vi "Setup.vi"(11 "Test Framework.lvclass":refnum<class "Test Framework.lvclass">) -> (0 "Error Out":errorcluster, 3 "Test Framework.lvclass Out":refnum<class "Test Framework.lvclass">)   [LabVIEW 2020, in "Test Framework.lvclass"]
uses:
  Test Framework.lvclass
  Path Control/PathControl.lvclass
  Instruments/Temperature Control/Temperature Control.lvclass
  Instruments/Power Supply/Power Supply.lvclass
  XML Handler/XML Handler.lvclass
  Test Framework.lvclass/Test Framework.ctl
  <vilib>/Utility/xml.llb/Read From XML File(string).vi
  Devices/Device.lvclass
  Measurements/Measurement.lvclass
panel:
  out "Available devices":string[](array[string])
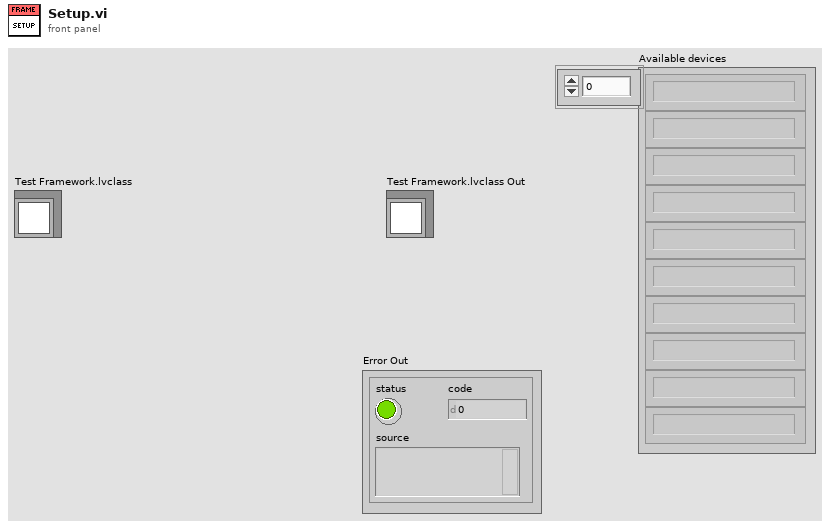
[diagram p1: front panel]
types:
  T1 = cluster{"Restart?":bool, "User system setting file":path}
  T2 = typedef "Device.lvclass/Device Information Cluster.ctl" = cluster{"Device Info":string[][], "Default Values":T3[], "Fetched info":string[][]}
  T3 = typedef "PIC-Device.lvclass/Register to Write.ctl" = cluster{"Register":u32, "Value":u32, "Dev Address":u32, "Physical Adress":u32}
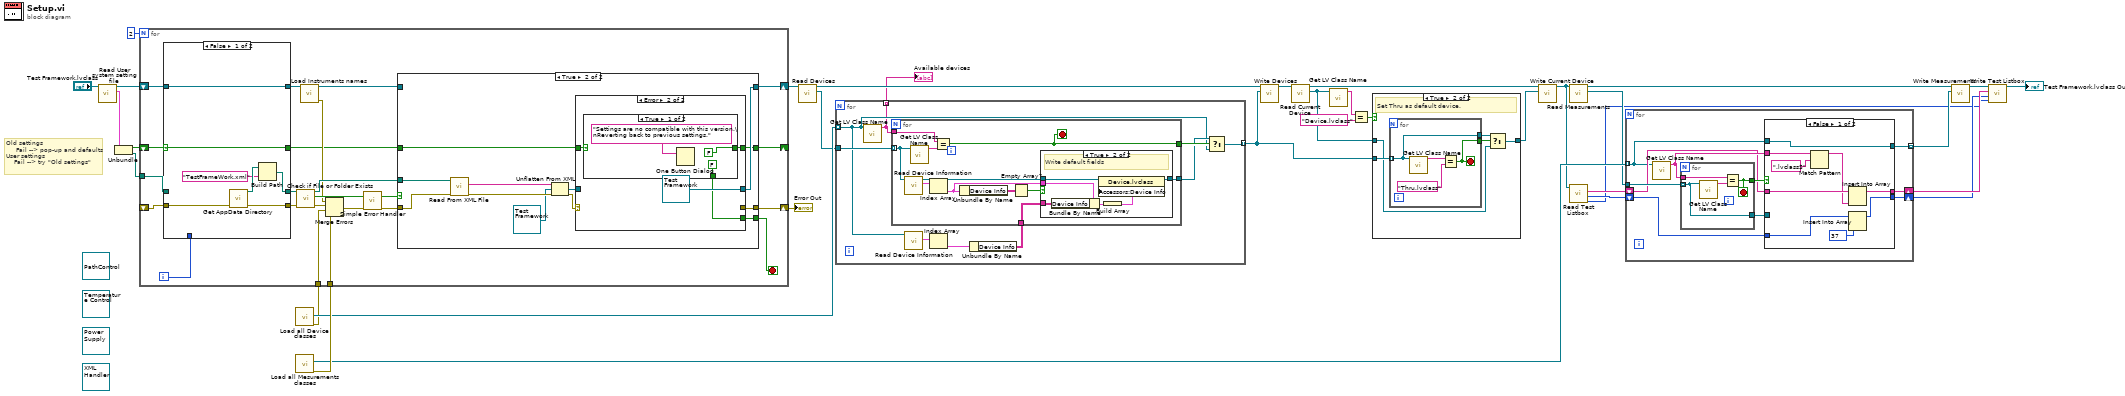
[diagram p0: block diagram]
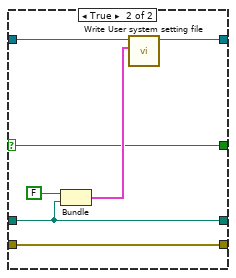
[diagram p2: hidden frame]
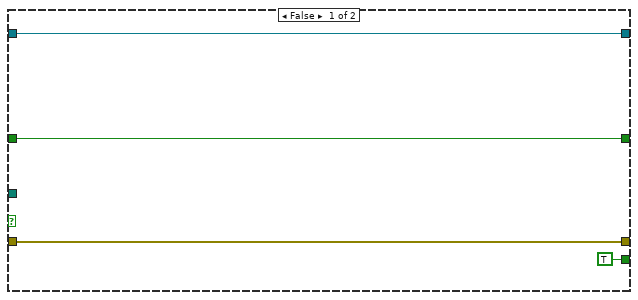
[diagram p3: hidden frame]
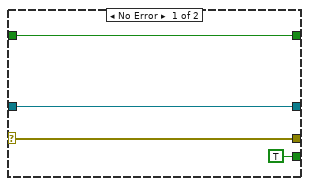
[diagram p4: hidden frame]
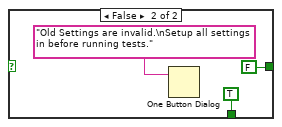
[diagram p5: hidden frame]
diagram:
  (unwired) refnum<class "XML Handler.lvclass"> refnum ("XML Handler.lvclass")
  (unwired) refnum<class "Power Supply.lvclass"> refnum ("Power Supply.lvclass")
  (unwired) refnum<class "Temperature Control.lvclass"> refnum ("Temperature Control.lvclass")
  (unwired) refnum<class "PathControl.lvclass"> refnum ("PathControl.lvclass")
  # "Old settings\n     Fail --> pop-up and defaults\nUser settings\n    Fail --> try \"Old settings\""
  n1 = call-dynamic "Read User system setting file.vi"("Test Framework in"="Test Framework.lvclass") -> ("User system setting file"=w6:T1, "Test Framework out"=w3:refnum<class "Test Framework.lvclass">)  [unwired: 9 in]
  n2 = Unbundle(w6) -> ("Restart?"=w5:bool, "User system setting file"=w4:path)
  n3 = call "Load all Device classes.vi"() -> ("Error Out"=w2:errorcluster, "Device Classes"=w19:refnum<class "Device.lvclass">[])  [unwired: 9 in, 1 out]
  n4 = call "Load all Mesurements classes.vi"() -> ("Error Out"=w34:errorcluster, "Measurement classes"=w29:refnum<class "Measurement.lvclass">[])  [unwired: 9 in, 1 out]
  n5 = for {
    N: 2 -> [_]
    tunnel: w34 -> [w51]
    tunnel: w4 -> [w44]
    shift-right: [w40] -> w20
    shift-left: _ -> [w39]
    shift-right: [w50] -> w33
    shift-left: w3 -> [w42]
    tunnel: w2 -> [w41]
    shift-right: [w37] -> _
    shift-left: w5 -> [w45]
    i -> [w35]
    stop <- w36 stop-if-true
    n6 = case shown="False" w45 {
      selector: w45 -> [w57 w64]
      tunnel: [w61 w68] -> w56
      tunnel: [w60 w65] -> w55
      tunnel: w44 -> [_ w68]
      tunnel: [w59 w69] -> w43
      tunnel: w42 -> [w59 w70]
      tunnel: w39 -> [w58 w65]
      tunnel: [w57 w64] -> w38
      tunnel: w35 -> [_ _]
      frame False {
        n7 = call "Get AppData Directory.vi"("Error In"=w58) -> ("Error Out"=w60:errorcluster, "Folder path"=w63:path)  [unwired: 8 in, 1 out]
        n8 = Build Path(base path=w63, name or relative path="TestFrameWork.xml") -> (appended path=w61:path)
      }
      frame True {
        n9 = Bundle(FALSE, "User system setting file"=w68) -> (w66:cluster{bool, "User system setting file":path})  [unwired: 1 in]
        n10 = call-dynamic "Write User system setting file.vi"("User system setting file"=w66, "Test Framework in"=w70) -> ("Test Framework out"=w69:refnum<class "Test Framework.lvclass">)  [unwired: 9 in]
      }
    }
    n11 = call <vilib>:"Check if File or Folder Exists.vi"("error in (no error)"=w55, "path"=w56) -> ("error out"=w53:errorcluster, "file or folder exists?"=w54:bool, "dup path"=w52:path)  [unwired: 7 in]
    n12 = call "Load Instruments names.vi"("Test Framework in"=w43) -> ("error out"=w48:errorcluster, "Test Framework out"=w49:refnum<class "Test Framework.lvclass">)  [unwired: 9 in]
    n13 = Merge Errors(w48, w53, w41, w51) -> (w47:errorcluster)
    n14 = call <vilib>:"Simple Error Handler.vi"("error in (no error)"=w47) -> ("error out"=w46:errorcluster)  [unwired: 4 in, 4 out]
    n15 = case shown="True" w54 {
      tunnel: w46 -> [w73 w86]
      tunnel: w52 -> [_ w85]
      tunnel: w49 -> [w74 _]
      tunnel: [w74 w80] -> w50
      tunnel: [w73 w79] -> w40
      tunnel: w38 -> [w72 w77]
      tunnel: [w72 w76] -> w37
      tunnel: [TRUE w75] -> w36
      frame False {
      }
      frame True {
        n16 = call-poly <vilib>:"Read From XML File.vi"("error in (no error)"=w86, "XML File Path"=w85) -> ("error out"=w83:errorcluster, "XML Elements"=w84:string)  [unwired: 7 in, 1 out]
        n17 = Unflatten From XML(xml string=w84, type=refnum<class "Test Framework.lvclass"> refnum ("Test Framework.lvclass"), error in (no error)=w83) -> (value=w81:refnum<class "Test Framework.lvclass">, error out=w78:errorcluster)
        n18 = case shown="Error" w78 {
          selector: w78 -> [w90 _]
          tunnel: w81 -> [w89 _]
          tunnel: [w89 refnum<class "Test Framework.lvclass"> refnum ("Test Framework.lvclass")] -> w80
          tunnel: [w90 _] -> w79
          tunnel: w77 -> [w88 w93]
          tunnel: [w88 w92] -> w76
          tunnel: [TRUE w91] -> w75
          frame No Error {
          }
          frame Error {
            n19 = case shown="True" w93 {
              tunnel: [FALSE FALSE] -> w92
              tunnel: [FALSE TRUE] -> w91
              frame True {
                n20 = One Button Dialog(message="Settings are no compatible with this version.\nReverting back to previous settings.") -> ()  [unwired: 1 in, 1 out]
              }
              frame False {
                n21 = One Button Dialog(message="Old Settings are invalid.\nSetup all settings in before running tests.") -> ()  [unwired: 1 in, 1 out]
              }
            }
          }
        }
      }
    }
  }
  "Error Out" <- w20
  n22 = call "Read Devices.vi"("Test Framework in"=w33) -> ("Devices"=w18:refnum<class "Device.lvclass">[], "Test Framework out"=w32:refnum<class "Test Framework.lvclass">)  [unwired: 9 in]
  n23 = for {
    tunnel: w19 -> [w102] mode=indexing
    tunnel: w18 -> [w109]
    tunnel: [w107] -> w13 mode=indexing
    tunnel: [w101] -> w8 mode=indexing
    n24 = call <vilib>:"Get LV Class Name.vi"("object"=w102) -> ("class name"=w101:string)  [unwired: 9 in, 1 out]
    n25 = call-dynamic "Read Device Information.vi"("Device in"=w102) -> ("Device Info"=w104:T2[])  [unwired: 8 in, 2 out]
    n26 = Index Array(array=w104) -> (element=w105:T2)  [unwired: 1 in]
    n27 = Unbundle By Name(w105) -> ("Device Info"=w103:string[][])
    n28 = for {
      tunnel: w109 -> [w116] mode=indexing
      tunnel: w101 -> [w119]
      tunnel: [w118] -> w108
      tunnel: [w113] -> w106
      tunnel: w103 -> [w111]
      stop <- w118 stop-if-true
      n29 = call-dynamic "Read Device Information.vi"("Device in"=w116) -> ("Device Info"=w117:T2[], "Device out"=w114:refnum<class "Device.lvclass">)  [unwired: 8 in, 1 out]
      n30 = call <vilib>:"Get LV Class Name.vi"("object"=w116) -> ("class name"=w120:string)  [unwired: 9 in, 1 out]
      n31 = Index Array(array=w117) -> (element=w112:T2)  [unwired: 1 in]
      n32 = Equal?(x=w119, y=w120) -> (x = y?=w118:bool)
      n33 = Unbundle By Name(w112) -> ("Device Info"=w115:string[][])
      n34 = Empty Array?(array=w115) -> (empty?=w110:bool)
      n35 = case shown="True" w110 {
        tunnel: w114 -> [w121 w127]
        tunnel: [w121 w126] -> w113
        tunnel: w112 -> [_ w125]
        tunnel: w111 -> [_ w122]
        frame False {
        }
        frame True {
          # "Write default fields"
          n36 = Bundle By Name(cluster=w125, "Device Info"=w122) -> (w124:T2)
          n37 = Build Array(w124) -> (w123:T2[])
          n38 = property class="Device.lvclass"(reference=w127, "Accessors:Device Info"=w123) -> (reference out=w126:refnum<class "Device.lvclass">)  [unwired: 1 in, 1 out]
        }
      }
    }
    n39 = Select(t=w106, s=w108, f=w102) -> (s? t:f=w107:refnum<class "Device.lvclass">)
  }
  "Available devices" <- w8
  n40 = call "Write Devices.vi"("Devices"=w13, "Test Framework in"=w32) -> ("Test Framework out"=w17:refnum<class "Test Framework.lvclass">)  [unwired: 9 in]
  n41 = call-dynamic "Read Current Device.vi"("Test Framework in"=w17) -> ("Current Device.lvclass"=w14:refnum<class "Device.lvclass">, "Test Framework out"=w15:refnum<class "Test Framework.lvclass">)  [unwired: 9 in]
  n42 = call <vilib>:"Get LV Class Name.vi"("object"=w14) -> ("class name"=w11:string)  [unwired: 9 in, 1 out]
  n43 = Equal?(x=w11, y="Device.lvclass") -> (x = y?=w10:bool)
  n44 = case shown="True" w10 {
    tunnel: w14 -> [w128 w130]
    tunnel: w13 -> [_ w133]
    tunnel: [w128 w129] -> w9
    frame False {
      # "Current device actual device. No changes."
    }
    frame True {
      # "Set Thru as default device."
      n45 = for {
        tunnel: w133 -> [w136] mode=indexing
        tunnel: [w136] -> w131
        tunnel: [w134] -> w132
        stop <- w134 stop-if-true
        n46 = call <vilib>:"Get LV Class Name.vi"("object"=w136) -> ("class name"=w135:string)  [unwired: 9 in, 1 out]
        n47 = Equal?(x=w135, y="Thru.lvclass") -> (x = y?=w134:bool)
      }
      n48 = Select(t=w131, s=w132, f=w130) -> (s? t:f=w129:refnum<class "Device.lvclass">)
    }
  }
  n49 = call-dynamic "Write Current Device.vi"("Current Device.lvclass"=w9, "Test Framework in"=w15) -> ("Test Framework out"=w16:refnum<class "Test Framework.lvclass">)  [unwired: 9 in]
  n50 = call "Read Measurements.vi"("Test Framework in"=w16) -> ("Measurements"=w28:refnum<class "Measurement.lvclass">[], "Test Framework out"=w27:refnum<class "Test Framework.lvclass">)  [unwired: 9 in]
  n51 = call "Read Test Listbox.vi"("Test Framework in"=w16) -> ("Value"=w21:i32, "Symbols"=w30:i32[], "Measurement Names"=w31:string[])  [unwired: 7 in, 1 out]
  n52 = for {
    tunnel: w29 -> [w138] mode=indexing
    tunnel: w28 -> [w147]
    shift-right: [w142] -> w23
    shift-left: w31 -> [w144]
    shift-right: [w141] -> w22
    shift-left: w30 -> [w143]
    tunnel: [w139] -> w26 mode=indexing
    n53 = call <vilib>:"Get LV Class Name.vi"("object"=w138) -> ("class name"=w145:string)  [unwired: 9 in, 1 out]
    n54 = for {
      tunnel: w147 -> [w161] mode=indexing
      tunnel: w145 -> [w160]
      tunnel: [w162] -> w146
      tunnel: [w161] -> w140
      stop <- w162 stop-if-true
      n55 = call <vilib>:"Get LV Class Name.vi"("object"=w161) -> ("class name"=w163:string)  [unwired: 9 in, 1 out]
      n56 = Equal?(x=w160, y=w163) -> (x = y?=w162:bool)
    }
    n57 = case shown="False" w146 {
      tunnel: w145 -> [w150 _]
      tunnel: w144 -> [w156 w158]
      tunnel: w143 -> [w154 w159]
      tunnel: [w155 w158] -> w142
      tunnel: [w152 w159] -> w141
      tunnel: w140 -> [_ w157]
      tunnel: [w151 w157] -> w139
      tunnel: w138 -> [w151 _]
      frame False {
        n58 = Match Pattern(string=w150, regular expression=".lvclass$") -> (before substring=w148:string)  [unwired: 1 in, 3 out]
        n59 = Insert Into Array(array=w156, new element=w148) -> (w155:string[])  [unwired: 1 in]
        n60 = Insert Into Array(array=w154, new element=37) -> (w152:i32[])  [unwired: 1 in]
      }
      frame True {
      }
    }
  }
  n61 = call "Write Measurements.vi"("Measurements"=w26, "Test Framework in"=w27) -> ("Test Framework out"=w25:refnum<class "Test Framework.lvclass">)  [unwired: 9 in]
  n62 = call "Write Test Listbox.vi"("Value"=w21, "Symbols"=w22, "Measurement Names"=w23, "Test Framework in"=w25) -> ("Test Framework out"=→"Test Framework.lvclass Out":refnum<class "Test Framework.lvclass">)  [unwired: 7 in]
